vi "rszvl_quotedInt_ReadCallback.vi"(5 "Attribute":T1={"Identifier"="", "Descriptive name"="", "Data Type"=enum."Integer 32", "Command"="", "Access"=2, "Range Table"="", "Read Callback"="", "Write Callback"="", "Range Callback"="", "Check Callback"="", "Rngtable Callback"="", "Coerce Callback"="", "Supported Models"="", "Instrument Options"="", "Repeated Capabilities"="", "Check Status Callback"="", "Index"=0, "Flag: OPC Wait"=FALSE, "Flag: Dont check status"=FALSE, "Flag: Cache Only"=FALSE} {"Access" items=["Read Only", "Write Only", "Read/Write"]}, 7 "Repeated Capability":string, 8 "error in":errorcluster, 11 "VISA resource name":refnum<visa-resource-name>) -> (0 "error out":errorcluster, 2 "Attribute Value I32":i32, 3 "VISA resource name out":refnum<visa-resource-name>)   [LabVIEW 2014]
uses:
  type_Attribute.ctl
  type_Attribute_Data_Type.ctl
  rszvl_rsidr_core.lvlib
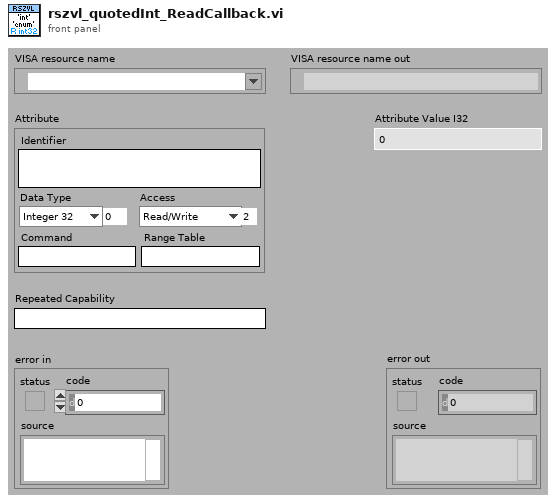
[diagram p1: front panel]
types:
  T1 = typedef "rszvl_rsidr_core.lvlib/type_Attribute.ctl" = cluster{"Identifier":string, "Descriptive name":string, "Data Type":T2, "Command":string, "Access":u16, "Range Table":string, "Read Callback":string, "Write Callback":string, "Range Callback":string, "Check Callback":string, "Rngtable Callback":string, "Coerce Callback":string, "Supported Models":string, "Instrument Options":string, "Repeated Capabilities":string, "Check Status Callback":string, "Index":i32, "Flag: OPC Wait":bool, "Flag: Dont check status":bool, "Flag: Cache Only":bool}
  T2 = typedef "rszvl_rsidr_core.lvlib/type_Attribute_Data_Type.ctl" = enum16{"Integer 32", "Double", "String", "Boolean", "None", "Integer 64"}
  T3 = typedef "rszvl_rsidr_core.lvlib/type_Session_Data.ctl" = cluster{"Instr type":string, "Instr type for err. msg.":string, "Installed Options":string[], "OPC Timeout":i32, "Query Instrument Status":bool, "Check Range":bool, "Check Options":bool, "Add LF to Write":bool, "Simulate":bool, "Logging":bool, "Logging params":variant, "Interface Type":enum16{"Unknown", "GPIB", "VXI", "GPIB_VXI", "ASRL", "PXI", "TCPIP", "USB", "SOCKET"}, "Fast Sweep":i32, "AdditionalFlags":i32, "WaitBeforeWrite":i32, "WaitBeforeRead":i32, "BinDataChunkSize":i64}
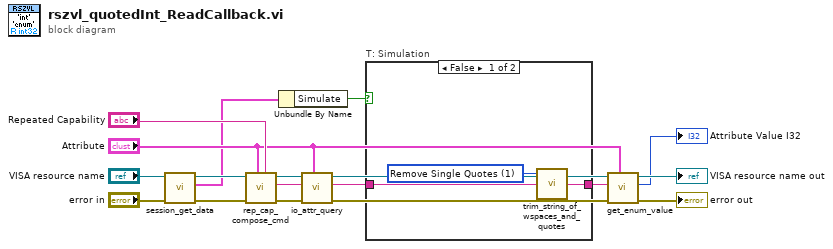
[diagram p0: block diagram]
diagram:
  n1 = call "session_get_data.vi"("error in"="error in", "VISA resource name"="VISA resource name") -> ("error out"=w6:errorcluster, "Session User Data out"=w2:T3, "VISA resource name out"=w5:refnum<visa-resource-name>)  [unwired: 7 in]
  n2 = call "rep_cap_compose_cmd.vi"("Repeated Capability"="Repeated Capability", "Attribute"="Attribute", "error in"=w6, "VISA resource name"=w5) -> ("error out"=w16:errorcluster, "Command out"=w17:string, "VISA resource name out"=w15:refnum<visa-resource-name>)  [unwired: 5 in]
  n3 = Unbundle By Name(w2) -> ("Simulate"=w1:bool)
  n4 = call "io_attr_query.vi"("Attribute"="Attribute", "error in"=w16, "write buffer"=w17, "VISA resource name"=w15) -> ("error out"=w14:errorcluster, "read buffer"=w4:string, "VISA resource name out"=w13:refnum<visa-resource-name>)  [unwired: 5 in]
  n5 = case "T: Simulation" shown="False" w1 {
    tunnel: w4 -> [w21 w22]
    tunnel: [w20 w22] -> w3
    frame False {
      w19 = u16 1 items=["Remove All Quotes", "Remove Single Quotes", "Remove Double Quotes", "Remove None"] ("Remove quotes (Remove All)")
      n6 = call "trim_string_of_wspaces_and_quotes.vi"("String in"=w21, "Remove quotes (Remove All)"=w19) -> ("String out"=w20:string)  [unwired: 3 in]
    }
    frame True {
    }
  }
  n7 = call "get_enum_value.vi"("Attribute"="Attribute", "error in"=w14, "String Value"=w3, "VISA resource name"=w13) -> ("error out"=→"error out":errorcluster, "I32 output"=→"Attribute Value I32":i32, "VISA resource name out"=→"VISA resource name out":refnum<visa-resource-name>)  [unwired: 5 in]
